vi "GetTimingSession.vi"(8 "error in (no error)":errorcluster, 11 "SyncPluginBase in":refnum<class "SyncPluginBase.lvclass">) -> (0 "error out":errorcluster, 2 "TimingSession":variant, 3 "SyncPluginBase out":refnum<class "SyncPluginBase.lvclass">)   [LabVIEW 2018, in "SyncPlugins.lvlib" / "SyncPluginBase.lvclass"]
uses:
  SyncPluginBase.lvclass
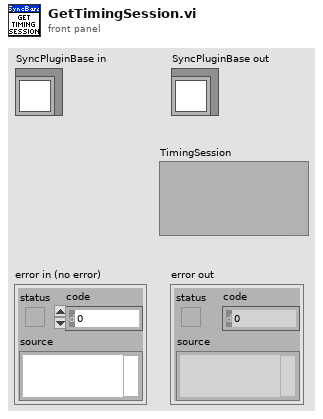
[diagram p1: front panel]
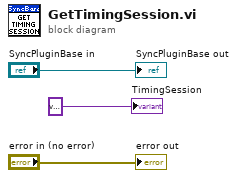
[diagram p0: block diagram]
diagram:
  "error out" <- "error in (no error)"
  "SyncPluginBase out" <- "SyncPluginBase in"
  "TimingSession" <- variant
